vi "as_loadParamList.vi"(4 "error in (no error)":errorcluster, 6 "Path In":path) -> (0 "error out":errorcluster, 2 "Path":path, 3 "Stimulus List":dbl[][](array[numeric]))   [LabVIEW 2009]
uses:
  <vilib>/Utility/file.llb/Read From Spreadsheet File (DBL).vi
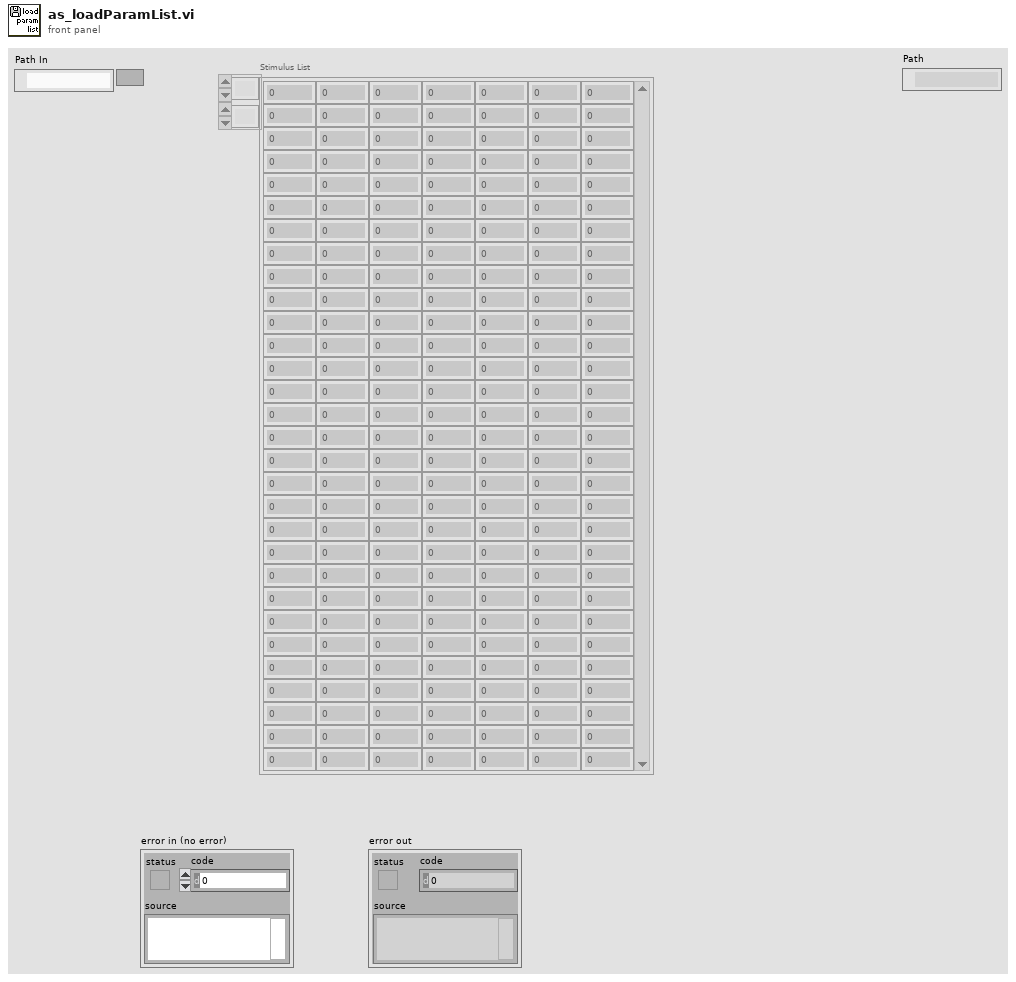
[diagram p1: front panel]
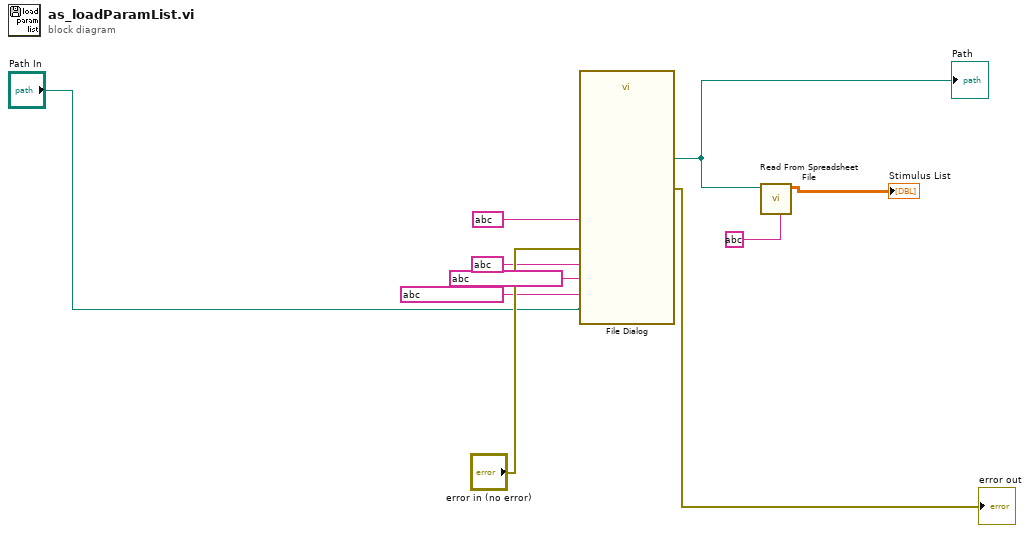
[diagram p0: block diagram]
diagram:
  n1 = call "File Dialog"("start path"="Path In", "prompt"=string ?, "button label"=string ?, "error in"="error in (no error)", "pattern (all files)"=string ?, "pattern label"=string ?) -> ("selected path"=w5:path, "error out"=→"error out":errorcluster)  [unwired: 6 in, 2 out]
  "Path" <- w5
  n2 = call-poly <vilib>:"Read From Spreadsheet File.vi"("delimiter (\\t)"=string ? ("delimiter (\\t)"), "file path (dialog if empty)"=w5) -> ("all rows"=→"Stimulus List":dbl[][])  [unwired: 5 in, 4 out]
